vi "Final4.0.vi"() -> ()   [LabVIEW 2022 SP3]
uses:
  <vilib>/DAQmx/read.llb/DAQmx Read (Digital Bool 1Line 1Point).vi
  <vilib>/DAQmx/write.llb/DAQmx Write (Digital Bool 1Line 1Point).vi
  <vilib>/DAQmx/read.llb/DAQmx Read (Analog DBL 1Chan 1Samp).vi
  <vilib>/DAQmx/create/channels.llb/DAQmx Create Channel (AI-Voltage-Basic).vi
  <vilib>/DAQmx/create/channels.llb/DAQmx Create Channel (DO-Digital Output).vi
  <vilib>/DAQmx/miscellaneous.llb/DAQmx Fill In Error Info.vi
  <vilib>/DAQmx/create/channels.llb/DAQmx Create Channel (DI-Digital Input).vi
panel:
  out "Weight":dbl
  in  "stop 2":bool
  in  "stop":bool
  out "IR 2":bool
  in  "IR Sensors 2":tag
  in  "VISA motor up off":refnum<visa-resource-name>
  out "Motor Up D L":bool
  in  "Motor Up 3":tag
  out "Motor Up L":bool
  in  "Motor Up":tag
  in  "VISA motor up on":refnum<visa-resource-name>
  in  "VISA Pump off":refnum<visa-resource-name>
  out "Pump off D L":bool
  out "Chamber off D L":bool
  in  "Pump Off":tag
  in  "Cham Off":tag
  out "Electrode L":bool
  in  "Electr":tag
  out "Pumb on L":bool
  in  "Pump On":tag
  in  "VISA Pump on on":refnum<visa-resource-name>
  out "Chamber on L":bool
  in  "Cham On":tag
  in  "VISA Motor down off":refnum<visa-resource-name>
  out "Motor down D L":bool
  in  "Motor down 4":tag
  out "Motor down L":bool
  in  "Motor down":tag
  in  "VISA Motor down on":refnum<visa-resource-name>
  out "IR L":bool
  in  "IR Sensors":tag
  out "Meter":dbl(knob) scale=0.0..10.0
  in  "y":dbl
  out "Pressure sensor":bool
  out "Weight Indicator":bool
  in  "Pressure Sen":tag
  in  "Weight indicator":tag
  in  "Weight Calibration":bool
  # "Weight Mesurement Dashboard"
  # "Indicators"
  # "Activation"
  # "Dectivation"
  # "Activation"
  # "Activation"
  # "Dectivation"
  # "Dectivation"
  # "Activation"
  # "Dectivation"
  # "Ports"
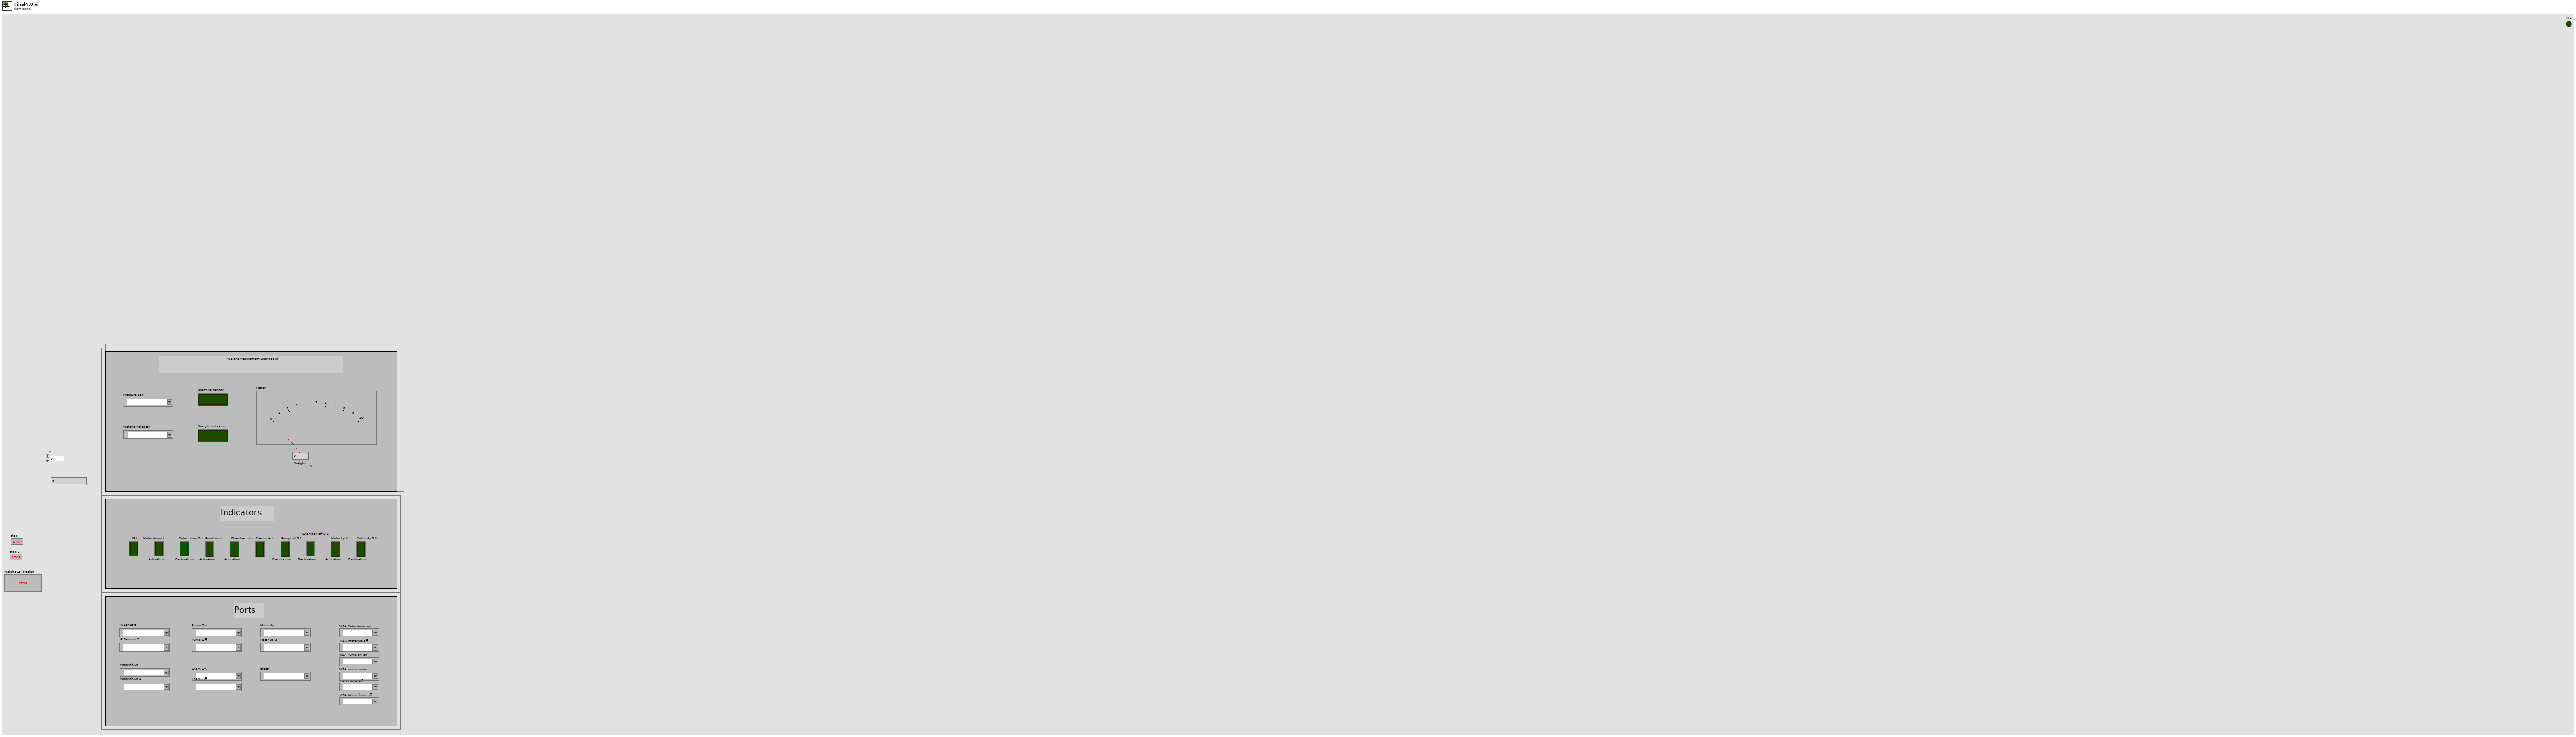
[diagram p1: front panel]
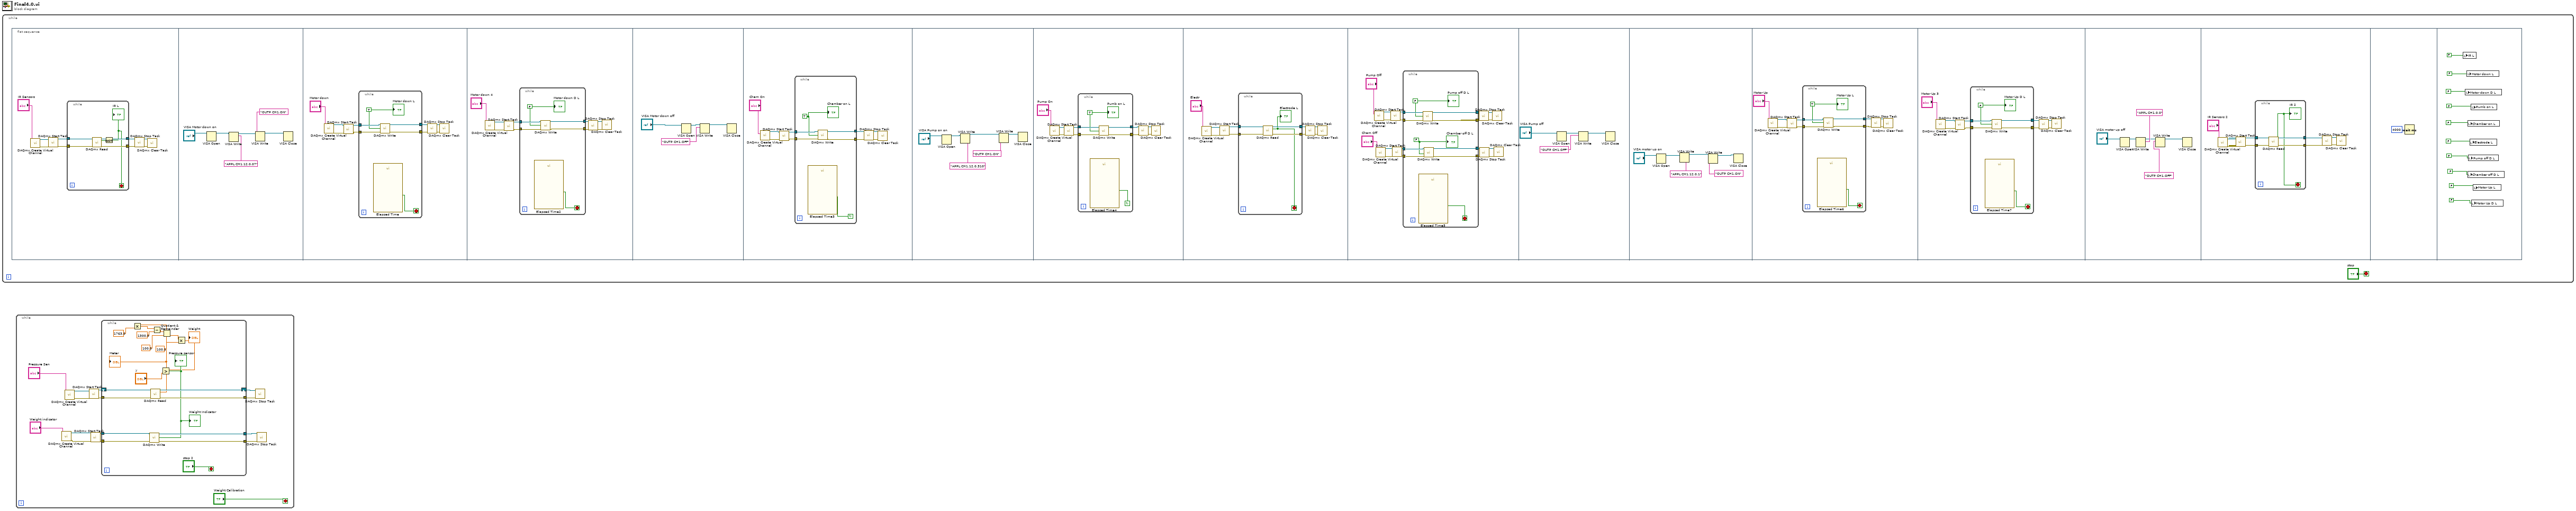
[diagram p0: block diagram]
diagram:
  n1 = while {
    stop <- "stop" stop-if-true
    n2 = flat-sequence {
      frame #0 {
        n3 = call-poly <vilib>:"DAQmx Create Virtual Channel.vi"("lines"="IR Sensors") -> ("task out"=w10:refnum<k21>, "error out"=w9:errorcluster)  [unwired: 13 in]
        n4 = call <vilib>:"DAQmx Start Task.vi"("task/channels in"=w10, "error in"=w9) -> ("task out"=w8:refnum<k21>, "error out"=w6:errorcluster)  [unwired: 12 in]
        n5 = while {
          tunnel: w8 -> [w16]
          tunnel: [w15] -> w7
          tunnel: w6 -> [w14]
          tunnel: [w13] -> w5
          stop <- w11 stop-if-true
          n6 = call-poly <vilib>:"DAQmx Read.vi"("task/channels in"=w16, "error in"=w14) -> ("task out"=w15:refnum<k21>, "data"=w12:bool, "error out"=w13:errorcluster)  [unwired: 11 in]
          n7 = Not(x=w12) -> (.not. x?=w11:bool)
          "IR L" <- w11
        }
        n8 = call <vilib>:"DAQmx Stop Task.vi"("task/channels in"=w7, "error in"=w5) -> ("task out"=w3:refnum<k21>, "error out"=w2:errorcluster)  [unwired: 12 in]
        n9 = call <vilib>:"DAQmx Clear Task.vi"("task in"=w3, "error in"=w2) -> ()  [unwired: 13 in, 1 out]
      }
      frame #1 {
        n10 = VISA Open(VISA resource name="VISA Motor down on") -> (VISA resource name=w19:refnum<visa-resource-name>)  [unwired: 4 in, 1 out]
        n11 = VISA Write(VISA resource name=w19, write buffer="APPL CH1,12,0.07") -> (VISA resource name out=w18:refnum<visa-resource-name>)  [unwired: 1 in, 2 out]
        n12 = VISA Write(VISA resource name=w18, write buffer="OUTP CH1,ON") -> (VISA resource name out=w17:refnum<visa-resource-name>)  [unwired: 1 in, 2 out]
        n13 = VISA Close(VISA resource name=w17) -> ()  [unwired: 1 in, 1 out]
      }
      frame #2 {
        n14 = call-poly <vilib>:"DAQmx Create Virtual Channel.vi"("lines"="Motor down") -> ("task out"=w28:refnum<k21>, "error out"=w27:errorcluster)  [unwired: 13 in]
        n15 = call <vilib>:"DAQmx Start Task.vi"("task/channels in"=w28, "error in"=w27) -> ("task out"=w31:refnum<k21>, "error out"=w29:errorcluster)  [unwired: 12 in]
        n16 = while {
          tunnel: w31 -> [w37]
          tunnel: [w36] -> w30
          tunnel: w29 -> [w35]
          tunnel: [w33] -> w26
          stop <- w32 stop-if-true
          w34 = TRUE
          n17 = call "Elapsed Time"() -> ("Time has Elapsed"=w32:bool)  [unwired: 12 in, 7 out]
          n18 = call-poly <vilib>:"DAQmx Write.vi"("task/channels in"=w37, "data"=w34, "error in"=w35) -> ("task out"=w36:refnum<k21>, "error out"=w33:errorcluster)  [unwired: 10 in, 1 out]
          "Motor down L" <- w34
        }
        n19 = call <vilib>:"DAQmx Stop Task.vi"("task/channels in"=w30, "error in"=w26) -> ("task out"=w24:refnum<k21>, "error out"=w23:errorcluster)  [unwired: 12 in]
        n20 = call <vilib>:"DAQmx Clear Task.vi"("task in"=w24, "error in"=w23) -> ()  [unwired: 13 in, 1 out]
      }
      frame #3 {
        n21 = call-poly <vilib>:"DAQmx Create Virtual Channel.vi"("lines"="Motor down 4") -> ("task out"=w43:refnum<k21>, "error out"=w42:errorcluster)  [unwired: 13 in]
        n22 = call <vilib>:"DAQmx Start Task.vi"("task/channels in"=w43, "error in"=w42) -> ("task out"=w46:refnum<k21>, "error out"=w44:errorcluster)  [unwired: 12 in]
        n23 = while {
          tunnel: w46 -> [w52]
          tunnel: [w51] -> w45
          tunnel: w44 -> [w50]
          tunnel: [w48] -> w41
          stop <- w47 stop-if-true
          w49 = FALSE
          n24 = call "Elapsed Time2"() -> ("Time has Elapsed"=w47:bool)  [unwired: 12 in, 7 out]
          n25 = call-poly <vilib>:"DAQmx Write.vi"("task/channels in"=w52, "data"=w49, "error in"=w50) -> ("task out"=w51:refnum<k21>, "error out"=w48:errorcluster)  [unwired: 10 in, 1 out]
          "Motor down D L" <- w49
        }
        n26 = call <vilib>:"DAQmx Stop Task.vi"("task/channels in"=w45, "error in"=w41) -> ("task out"=w39:refnum<k21>, "error out"=w38:errorcluster)  [unwired: 12 in]
        n27 = call <vilib>:"DAQmx Clear Task.vi"("task in"=w39, "error in"=w38) -> ()  [unwired: 13 in, 1 out]
      }
      frame #4 {
        n28 = VISA Open(VISA resource name="VISA Motor down off") -> (VISA resource name=w55:refnum<visa-resource-name>)  [unwired: 4 in, 1 out]
        n29 = VISA Write(VISA resource name=w55, write buffer="OUTP CH1,OFF") -> (VISA resource name out=w56:refnum<visa-resource-name>)  [unwired: 1 in, 2 out]
        n30 = VISA Close(VISA resource name=w56) -> ()  [unwired: 1 in, 1 out]
      }
      frame #5 {
        n31 = call-poly <vilib>:"DAQmx Create Virtual Channel.vi"("lines"="Cham On") -> ("task out"=w62:refnum<k21>, "error out"=w61:errorcluster)  [unwired: 13 in]
        n32 = call <vilib>:"DAQmx Start Task.vi"("task/channels in"=w62, "error in"=w61) -> ("task out"=w65:refnum<k21>, "error out"=w63:errorcluster)  [unwired: 12 in]
        n33 = while {
          tunnel: w65 -> [w71]
          tunnel: [w70] -> w64
          tunnel: w63 -> [w69]
          tunnel: [w67] -> w60
          stop <- w66 continue-if-true
          w68 = TRUE
          n34 = call "Elapsed Time3"() -> ("Time has Elapsed"=w66:bool)  [unwired: 12 in, 7 out]
          n35 = call-poly <vilib>:"DAQmx Write.vi"("task/channels in"=w71, "data"=w68, "error in"=w69) -> ("task out"=w70:refnum<k21>, "error out"=w67:errorcluster)  [unwired: 10 in, 1 out]
          "Chamber on L" <- w68
        }
        n36 = call <vilib>:"DAQmx Stop Task.vi"("task/channels in"=w64, "error in"=w60) -> ("task out"=w58:refnum<k21>, "error out"=w57:errorcluster)  [unwired: 12 in]
        n37 = call <vilib>:"DAQmx Clear Task.vi"("task in"=w58, "error in"=w57) -> ()  [unwired: 13 in, 1 out]
      }
      frame #6 {
        n38 = VISA Open(VISA resource name="VISA Pump on on") -> (VISA resource name=w74:refnum<visa-resource-name>)  [unwired: 4 in, 1 out]
        n39 = VISA Write(VISA resource name=w74, write buffer="APPL CH1,12,0.310") -> (VISA resource name out=w73:refnum<visa-resource-name>)  [unwired: 1 in, 2 out]
        n40 = VISA Write(VISA resource name=w73, write buffer="OUTP CH1,ON") -> (VISA resource name out=w72:refnum<visa-resource-name>)  [unwired: 1 in, 2 out]
        n41 = VISA Close(VISA resource name=w72) -> ()  [unwired: 1 in, 1 out]
      }
      frame #7 {
        n42 = call-poly <vilib>:"DAQmx Create Virtual Channel.vi"("lines"="Pump On") -> ("task out"=w86:refnum<k21>, "error out"=w85:errorcluster)  [unwired: 13 in]
        n43 = call <vilib>:"DAQmx Start Task.vi"("task/channels in"=w86, "error in"=w85) -> ("task out"=w84:refnum<k21>, "error out"=w83:errorcluster)  [unwired: 12 in]
        n44 = while {
          tunnel: w84 -> [w92]
          tunnel: w83 -> [w91]
          tunnel: [w90] -> w82
          tunnel: [w89] -> w81
          stop <- w87 continue-if-true
          w88 = TRUE
          n45 = call "Elapsed Time4"() -> ("Time has Elapsed"=w87:bool)  [unwired: 12 in, 7 out]
          n46 = call-poly <vilib>:"DAQmx Write.vi"("task/channels in"=w92, "data"=w88, "error in"=w91) -> ("task out"=w90:refnum<k21>, "error out"=w89:errorcluster)  [unwired: 10 in, 1 out]
          "Pumb on L" <- w88
        }
        n47 = call <vilib>:"DAQmx Stop Task.vi"("task/channels in"=w82, "error in"=w81) -> ("task out"=w79:refnum<k21>, "error out"=w78:errorcluster)  [unwired: 12 in]
        n48 = call <vilib>:"DAQmx Clear Task.vi"("task in"=w79, "error in"=w78) -> ()  [unwired: 13 in, 1 out]
      }
      frame #8 {
        n49 = call-poly <vilib>:"DAQmx Create Virtual Channel.vi"("lines"="Electr") -> ("task out"=w101:refnum<k21>, "error out"=w100:errorcluster)  [unwired: 13 in]
        n50 = call <vilib>:"DAQmx Start Task.vi"("task/channels in"=w101, "error in"=w100) -> ("task out"=w99:refnum<k21>, "error out"=w97:errorcluster)  [unwired: 12 in]
        n51 = while {
          tunnel: w99 -> [w106]
          tunnel: [w105] -> w98
          tunnel: w97 -> [w104]
          tunnel: [w103] -> w96
          stop <- w102 stop-if-true
          n52 = call-poly <vilib>:"DAQmx Read.vi"("task/channels in"=w106, "error in"=w104) -> ("task out"=w105:refnum<k21>, "data"=w102:bool, "error out"=w103:errorcluster)  [unwired: 11 in]
          "Electrode L" <- w102
        }
        n53 = call <vilib>:"DAQmx Stop Task.vi"("task/channels in"=w98, "error in"=w96) -> ("task out"=w94:refnum<k21>, "error out"=w93:errorcluster)  [unwired: 12 in]
        n54 = call <vilib>:"DAQmx Clear Task.vi"("task in"=w94, "error in"=w93) -> ()  [unwired: 13 in, 1 out]
      }
      frame #9 {
        n55 = call-poly <vilib>:"DAQmx Create Virtual Channel.vi"("lines"="Pump Off") -> ("task out"=w124:refnum<k21>, "error out"=w121:errorcluster)  [unwired: 13 in]
        n56 = call-poly <vilib>:"DAQmx Create Virtual Channel.vi"("lines"="Cham Off") -> ("task out"=w118:refnum<k21>, "error out"=w117:errorcluster)  [unwired: 13 in]
        n57 = call <vilib>:"DAQmx Start Task.vi"("task/channels in"=w124, "error in"=w121) -> ("task out"=w123:refnum<k21>, "error out"=w120:errorcluster)  [unwired: 12 in]
        n58 = call <vilib>:"DAQmx Start Task.vi"("task/channels in"=w118, "error in"=w117) -> ("task out"=w116:refnum<k21>, "error out"=w115:errorcluster)  [unwired: 12 in]
        n59 = while {
          tunnel: w123 -> [w135]
          tunnel: [w134] -> w122
          tunnel: w120 -> [w133]
          tunnel: [w132] -> w119
          tunnel: w116 -> [w130]
          tunnel: w115 -> [w129]
          tunnel: [w128] -> w111
          tunnel: [w127] -> w114
          stop <- w125 stop-if-true
          w126 = FALSE
          w131 = FALSE
          n60 = call "Elapsed Time5"() -> ("Time has Elapsed"=w125:bool)  [unwired: 12 in, 7 out]
          n61 = call-poly <vilib>:"DAQmx Write.vi"("task/channels in"=w135, "data"=w131, "error in"=w133) -> ("task out"=w134:refnum<k21>, "error out"=w132:errorcluster)  [unwired: 10 in, 1 out]
          n62 = call-poly <vilib>:"DAQmx Write.vi"("task/channels in"=w130, "data"=w126, "error in"=w129) -> ("task out"=w127:refnum<k21>, "error out"=w128:errorcluster)  [unwired: 10 in, 1 out]
          "Pump off D L" <- w131
          "Chamber off D L" <- w126
        }
        n63 = call <vilib>:"DAQmx Stop Task.vi"("task/channels in"=w122, "error in"=w119) -> ("task out"=w110:refnum<k21>, "error out"=w109:errorcluster)  [unwired: 12 in]
        n64 = call <vilib>:"DAQmx Stop Task.vi"("task/channels in"=w114, "error in"=w111) -> ("task out"=w108:refnum<k21>, "error out"=w107:errorcluster)  [unwired: 12 in]
        n65 = call <vilib>:"DAQmx Clear Task.vi"("task in"=w110, "error in"=w109) -> ()  [unwired: 13 in, 1 out]
        n66 = call <vilib>:"DAQmx Clear Task.vi"("task in"=w108, "error in"=w107) -> ()  [unwired: 13 in, 1 out]
      }
      frame #10 {
        n67 = VISA Open(VISA resource name="VISA Pump off") -> (VISA resource name=w138:refnum<visa-resource-name>)  [unwired: 4 in, 1 out]
        n68 = VISA Write(VISA resource name=w138, write buffer="OUTP CH1,OFF") -> (VISA resource name out=w137:refnum<visa-resource-name>)  [unwired: 1 in, 2 out]
        n69 = VISA Close(VISA resource name=w137) -> ()  [unwired: 1 in, 1 out]
      }
      frame #11 {
        n70 = VISA Open(VISA resource name="VISA motor up on") -> (VISA resource name=w142:refnum<visa-resource-name>)  [unwired: 4 in, 1 out]
        n71 = VISA Write(VISA resource name=w142, write buffer="APPL CH1,12,0.1") -> (VISA resource name out=w141:refnum<visa-resource-name>)  [unwired: 1 in, 2 out]
        n72 = VISA Write(VISA resource name=w141, write buffer="OUTP CH1,ON") -> (VISA resource name out=w140:refnum<visa-resource-name>)  [unwired: 1 in, 2 out]
        n73 = VISA Close(VISA resource name=w140) -> ()  [unwired: 1 in, 1 out]
      }
      frame #12 {
        n74 = call-poly <vilib>:"DAQmx Create Virtual Channel.vi"("lines"="Motor Up") -> ("task out"=w151:refnum<k21>, "error out"=w150:errorcluster)  [unwired: 13 in]
        n75 = call <vilib>:"DAQmx Start Task.vi"("task/channels in"=w151, "error in"=w150) -> ("task out"=w154:refnum<k21>, "error out"=w152:errorcluster)  [unwired: 12 in]
        n76 = while {
          tunnel: w154 -> [w160]
          tunnel: [w159] -> w153
          tunnel: w152 -> [w158]
          tunnel: [w156] -> w149
          stop <- w155 stop-if-true
          w157 = TRUE
          n77 = call "Elapsed Time6"() -> ("Time has Elapsed"=w155:bool)  [unwired: 12 in, 7 out]
          n78 = call-poly <vilib>:"DAQmx Write.vi"("task/channels in"=w160, "data"=w157, "error in"=w158) -> ("task out"=w159:refnum<k21>, "error out"=w156:errorcluster)  [unwired: 10 in, 1 out]
          "Motor Up L" <- w157
        }
        n79 = call <vilib>:"DAQmx Stop Task.vi"("task/channels in"=w153, "error in"=w149) -> ("task out"=w147:refnum<k21>, "error out"=w146:errorcluster)  [unwired: 12 in]
        n80 = call <vilib>:"DAQmx Clear Task.vi"("task in"=w147, "error in"=w146) -> ()  [unwired: 13 in, 1 out]
      }
      frame #13 {
        n81 = call-poly <vilib>:"DAQmx Create Virtual Channel.vi"("lines"="Motor Up 3") -> ("task out"=w166:refnum<k21>, "error out"=w165:errorcluster)  [unwired: 13 in]
        n82 = call <vilib>:"DAQmx Start Task.vi"("task/channels in"=w166, "error in"=w165) -> ("task out"=w169:refnum<k21>, "error out"=w167:errorcluster)  [unwired: 12 in]
        n83 = while {
          tunnel: w169 -> [w175]
          tunnel: [w174] -> w168
          tunnel: w167 -> [w173]
          tunnel: [w171] -> w164
          stop <- w170 stop-if-true
          w172 = FALSE
          n84 = call "Elapsed Time7"() -> ("Time has Elapsed"=w170:bool)  [unwired: 12 in, 7 out]
          n85 = call-poly <vilib>:"DAQmx Write.vi"("task/channels in"=w175, "data"=w172, "error in"=w173) -> ("task out"=w174:refnum<k21>, "error out"=w171:errorcluster)  [unwired: 10 in, 1 out]
          "Motor Up D L" <- w172
        }
        n86 = call <vilib>:"DAQmx Stop Task.vi"("task/channels in"=w168, "error in"=w164) -> ("task out"=w162:refnum<k21>, "error out"=w161:errorcluster)  [unwired: 12 in]
        n87 = call <vilib>:"DAQmx Clear Task.vi"("task in"=w162, "error in"=w161) -> ()  [unwired: 13 in, 1 out]
      }
      frame #14 {
        n88 = VISA Open(VISA resource name="VISA motor up off") -> (VISA resource name=w177:refnum<visa-resource-name>)  [unwired: 4 in, 1 out]
        n89 = VISA Write(VISA resource name=w177, write buffer="APPL CH1,0,0") -> (VISA resource name out=w176:refnum<visa-resource-name>)  [unwired: 1 in, 2 out]
        n90 = VISA Write(VISA resource name=w176, write buffer="OUTP CH1,OFF") -> (VISA resource name out=w180:refnum<visa-resource-name>)  [unwired: 1 in, 2 out]
        n91 = VISA Close(VISA resource name=w180) -> ()  [unwired: 1 in, 1 out]
      }
      frame #15 {
        n92 = call-poly <vilib>:"DAQmx Create Virtual Channel.vi"("lines"="IR Sensors 2") -> ("task out"=w190:refnum<k21>, "error out"=w189:errorcluster)  [unwired: 13 in]
        n93 = call <vilib>:"DAQmx Start Task.vi"("task/channels in"=w190, "error in"=w189) -> ("task out"=w188:refnum<k21>, "error out"=w186:errorcluster)  [unwired: 12 in]
        n94 = while {
          tunnel: w188 -> [w195]
          tunnel: [w194] -> w187
          tunnel: w186 -> [w193]
          tunnel: [w192] -> w185
          stop <- w191 stop-if-true
          n95 = call-poly <vilib>:"DAQmx Read.vi"("task/channels in"=w195, "error in"=w193) -> ("task out"=w194:refnum<k21>, "data"=w191:bool, "error out"=w192:errorcluster)  [unwired: 11 in]
          "IR 2" <- w191
        }
        n96 = call <vilib>:"DAQmx Stop Task.vi"("task/channels in"=w187, "error in"=w185) -> ("task out"=w183:refnum<k21>, "error out"=w182:errorcluster)  [unwired: 12 in]
        n97 = call <vilib>:"DAQmx Clear Task.vi"("task in"=w183, "error in"=w182) -> ()  [unwired: 13 in, 1 out]
      }
      frame #16 {
        n98 = Wait (ms)(milliseconds to wait=u32 4000) -> ()  [unwired: 1 out]
      }
      frame #17 {
        n99 = local write "IR L"(FALSE) -> ()
        n100 = local write "Motor down D L"(FALSE) -> ()
        n101 = local write "Motor down L"(FALSE) -> ()
        n102 = local write "Chamber on L"(FALSE) -> ()
        n103 = local write "Chamber off D L"(FALSE) -> ()
        n104 = local write "Pump off D L"(FALSE) -> ()
        n105 = local write "Electrode L"(FALSE) -> ()
        n106 = local write "Pumb on L"(FALSE) -> ()
        n107 = local write "Motor Up D L"(FALSE) -> ()
        n108 = local write "Motor Up L"(FALSE) -> ()
      }
    }
  }
  n109 = while {
    stop <- "Weight Calibration" stop-if-true
    n110 = call-poly <vilib>:"DAQmx Create Virtual Channel.vi"("lines"="Weight indicator") -> ("task out"=w216:refnum<k21>, "error out"=w213:errorcluster)  [unwired: 13 in]
    n111 = call-poly <vilib>:"DAQmx Create Virtual Channel.vi"("physical channels"="Pressure Sen") -> ("task out"=w221:refnum<k21>, "error out"=w212:errorcluster)  [unwired: 13 in]
    n112 = call <vilib>:"DAQmx Start Task.vi"("task/channels in"=w221, "error in"=w212) -> ("task out"=w220:refnum<k21>, "error out"=w210:errorcluster)  [unwired: 12 in]
    n113 = call <vilib>:"DAQmx Start Task.vi"("task/channels in"=w216, "error in"=w213) -> ("task out"=w215:refnum<k21>, "error out"=w209:errorcluster)  [unwired: 12 in]
    n114 = while {
      shift-right: [w240] -> w219
      shift-left: w220 -> [w241]
      tunnel: w215 -> [w239]
      tunnel: [w238] -> w214
      tunnel: [w237] -> w211
      tunnel: w210 -> [w236]
      tunnel: w209 -> [w235]
      tunnel: [w234] -> w208
      stop <- "stop 2" stop-if-true
      n115 = call-poly <vilib>:"DAQmx Read.vi"("task/channels in"=w241, "error in"=w236) -> ("task out"=w240:refnum<k21>, "data"=w224:dbl, "error out"=w237:errorcluster)  [unwired: 11 in]
      "Meter" <- w224
      n116 = Multiply(x=w224, y=1763.0) -> (x*y=w228:dbl)
      n117 = Subtract(x=w228, y=1300.0) -> (x-y=w225:dbl)
      n118 = Quotient & Remainder(x=w225, y=100.0) -> (floor(x/y)=w231:dbl)  [unwired: 1 out]
      n119 = Multiply(x=w231, y=100.0) -> (x*y=w223:dbl)
      "Weight" <- w223
      n120 = Greater?(x=w223, y="y") -> (0:w233:bool)
      "Pressure sensor" <- w233
      "Weight Indicator" <- w233
      n121 = call-poly <vilib>:"DAQmx Write.vi"("task/channels in"=w239, "data"=w233, "error in"=w235) -> ("task out"=w238:refnum<k21>, "error out"=w234:errorcluster)  [unwired: 10 in, 1 out]
    }
    n122 = call <vilib>:"DAQmx Stop Task.vi"("task/channels in"=w219, "error in"=w211) -> ()  [unwired: 12 in, 2 out]
    n123 = call <vilib>:"DAQmx Stop Task.vi"("task/channels in"=w214, "error in"=w208) -> ()  [unwired: 12 in, 2 out]
  }
